vi "Set graph range.vi"(6 "Data In":T4, 9 "Timeline":T9, 10 "Xinformation Out in":T1, 11 "XYGraph in":T3) -> (0 "error out":errorcluster, 2 "Xinformation Out out":T1)   [LabVIEW 2017, in "XGrapher.xctl"]
uses:
  XGrapher.xctl
  Typedefs/Xctrl-Timeline graph ref.ctl
  Data 1.ctl
  Typedefs/Xctrl-Data array.ctl
  Typedefs/Xcrtl-Data format definition.ctl
  Typedefs/Xctl-XY data type definition.ctl
  Typedefs/Xctrl-ROI type enum.ctl
  Typedefs/Xctrl-Waveform graph ref.ctl
  Typedefs/Xinformation.ctl
  Typedefs/Xcrtl-Click Operation.ctl
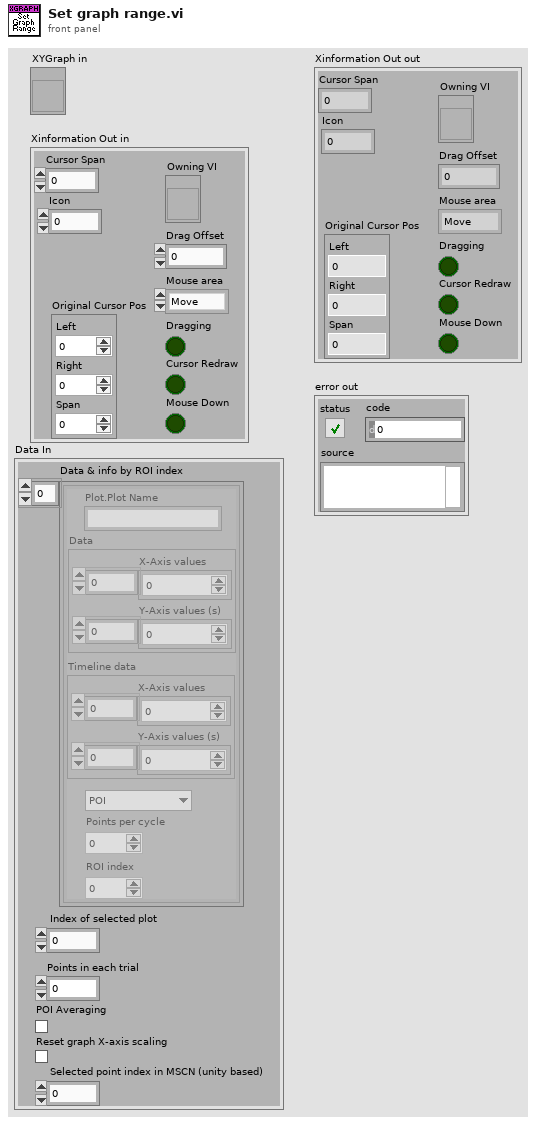
[diagram p1: front panel]
types:
  T1 = typedef "XGrapher.xctl/Xinformation.ctl" = cluster{"Cursor Span":dbl, "Icon":u16, "Mouse Down":bool, "Owning VI":refnum<vi>, "Mouse area":T2, "Dragging":bool, "Drag Offset":dbl, "Original Cursor Pos":cluster{"Left":dbl, "Right":dbl, "Span":dbl}, "Cursor Redraw":bool}
  T2 = typedef "XGrapher.xctl/Xcrtl-Click Operation.ctl" = enum16{"Move", "left cursor", "right cursor", "none"}
  T3 = typedef "XGrapher.xctl/Xctrl-Waveform graph ref.ctl" = refnum<vi>
  T4 = typedef "XGrapher.xctl/Data 1.ctl" = cluster{"Data & info by ROI index":T5, "Index of selected plot":u16, "Points in each trial":i32, "POI Averaging":bool, "Reset graph X-axis scaling":bool, "Selected point index in MSCN (unity based)":u16}
  T5 = typedef "Xctrl-Data array.ctl" = T6[]
  T6 = typedef "XGrapher.xctl/Xcrtl-Data format definition.ctl" = cluster{"Plot.Plot Name":string, "Data":T7, "Timeline data":T7, "Type":T8, "Points per cycle":u16, "ROI index":u16}
  T7 = typedef "XGrapher.xctl/Xctl-XY data type definition.ctl" = cluster{"X-Axis values":sgl[], "Y-Axis values (s)":sgl[]}
  T8 = typedef "Xctrl-ROI type enum.ctl" = enum16{"POI", "Mini-scan", "Group"}
  T9 = typedef "XGrapher.xctl/Xctrl-Timeline graph ref.ctl" = refnum<vi>
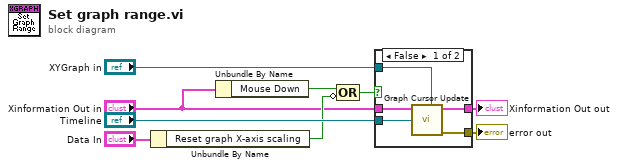
[diagram p0: block diagram]
diagram:
  n1 = Unbundle By Name("Data In") -> ("Reset graph X-axis scaling"=w7:bool)
  n2 = Unbundle By Name("Xinformation Out in") -> ("Mouse Down"=w5:bool)
  n3 = Compound Arithmetic op=OR(w5, invert w7) -> (w6:bool)
  n4 = case shown="False" w6 {
    tunnel: "Timeline" -> [w14 _]
    tunnel: [w13 w15] -> w2
    tunnel: "XYGraph in" -> [w10 _]
    tunnel: [w12 _] -> w3
    tunnel: "Xinformation Out in" -> [w11 w15]
    frame False {
      n5 = call "Graph Cursor Update.vi"("Waveform Ref in"=w10, "Timeline Ref in"=w14, "Xinformation In"=w11) -> ("error out"=w12:errorcluster, "Xinformation Out"=w13:T1)  [unwired: 6 in, 1 out]
    }
    frame True {
    }
  }
  "error out" <- w3
  "Xinformation Out out" <- w2
